vi "Camber controller instrument on-off capability.vi"() -> ()   [LabVIEW 2014]
uses:
  <vilib>/Instr/_visa.llb/VISA Configure Serial Port (Instr).vi
  <vilib>/Utility/file.llb/Write To Spreadsheet File (string).vi
  <vilib>/Utility/file.llb/Read From Spreadsheet File (string).vi
  Environmental Chamber LabVIEW and Instruments/Drivers and Software/Keithley 2100 Series/Public/Configure/Configure 2 Wire Resistance.vi
  Environmental Chamber LabVIEW and Instruments/Drivers and Software/keithley_6430/Keithley 6430/Keithley 6430.lvlib
  Environmental Chamber LabVIEW and Instruments/Drivers and Software/keithley_24xx/Keithley 24XX/Keithley 24XX.lvlib
  Environmental Chamber LabVIEW and Instruments/Drivers and Software/Keithley 2100 Series/Keithley 2100 Series.lvlib
panel:
  out "Arduino QCM freq":T1 caption="Arduino\nQCM freq" {"QCM1" format="%#_8g"; "QCM2" format="%#_8g"; "QCM3" format="%#_8g"; "QCM4" format="%#_8g"; "QCM5" format="%#_8g"}
  in  "Stop":bool
  out "Currently saving data":bool
  in  "Tab Control":T2(tab)
  in  "Instrument Addresses":T3={"J-KEM"="COM3", "Keithley-6430"="GPIB0::30::INSTR", "Keithley-2420"="GPIB1::24::INSTR", "Keithley-2100"="K-2100", "SRS-QCM200"="COM6", "ArduinoQCM1"="COM21", "ArduinoQCM2"="COM22", "ArduinoQCM3"="COM23", "ArduinoQCM4"="COM24", "ArduinoQCM5"="COM26"}
  in  "Instrument on/off":T4
  in  "Data logging settings":T5={"Save during sequence only"=TRUE, "Save now"=FALSE, "seconds between\ndata points"=0.0, "Current data file path"=path "", "Save sample names"={"QCM1"="aQCM2", "QCM2"="aQCM2", "QCM3"="aQCM3", "QCM4"="aQCM4", "QCM5"="aQCM5", "QCM6"="aQCM6", "SRS"="sample_SRS", "K-2420"="Keithley2420", "K-6430"="Keithley6430", "K-2100"="Keithley2100"}, "Experiment Notes"=""} {"seconds between\ndata points" min=0.0 max=30.0 format="%#_13g"}
  out "Sequence\npreview":cluster{dbl[], dbl[]}[](graph) caption="Sequence preview"
  in  "Pressure control cluster":T6={"Save sequence"=FALSE, "Clear sequence"=FALSE, "Import sequence file"=FALSE, "Tare elapsed time"=TRUE, "Run Sequence"=FALSE, "Stop program when sequence ends"=TRUE, "User-defined\nsequence"=[], "Sequence end time"=""} caption="Sequence settings"
  in  "Pressure parameters cluster":T7={"valve % open"=100.0, "Desired pressure"=0.0, "Vapor sccm"=0.0, "Gas sccm"=0.0, "Valve mode"=enum."% Open", "Pressure Mode"=enum."Abs. pressure", "analyte partial pressure"=100.0, "Turbo pump\nauto on"=TRUE, "Valve position (%)"=0.0, "read pressure"=0.0, "read vapor flow"=0.0, "read gas flow"=0.0} caption="Pressure settings" {"read gas flow" format="%#_3g"; "read vapor flow" format="%#_3g"; "read pressure" format="%#_7f"; "Valve position (%)" format="%#_3g"; "analyte partial pressure" min=0.0 max=100.0 step=5.0; "Gas sccm" min=0 max=200 step=5; "Vapor sccm" min=0 max=200 step=5; "Desired pressure" min=0.0 max=760.0 step=5.0; "valve % open" min=0.0 max=100.0 step=5.0 format="%#_2f"}
  out "Pressure chart":dbl(graph)
  out "Temp chart":dbl(graph)
  in  "SRS cluster":T8={"QCM plot"={"Numeric Control"=0.0, "Resistance out"=0.0}, "Gate time (sec)"=1, "Freq (MHz)"=0.0, "Tare mass"=FALSE} caption="SRS QCM" {"Freq (MHz)" format="%.6f"; "Gate time (sec)" items=["0.1 seconds", "1.0 seconds", "10.0 seconds"]}
  out "Keithley charts cluster":T9 caption="Keithley measurements"
  in  "Clear all charts":bool
  out "Elapsed time (min)":dbl
  out "State date/time":string caption="Start time"
  out "Arduino QCM plots":T10 caption="Arduino/OpenQCM"
  # "100%"
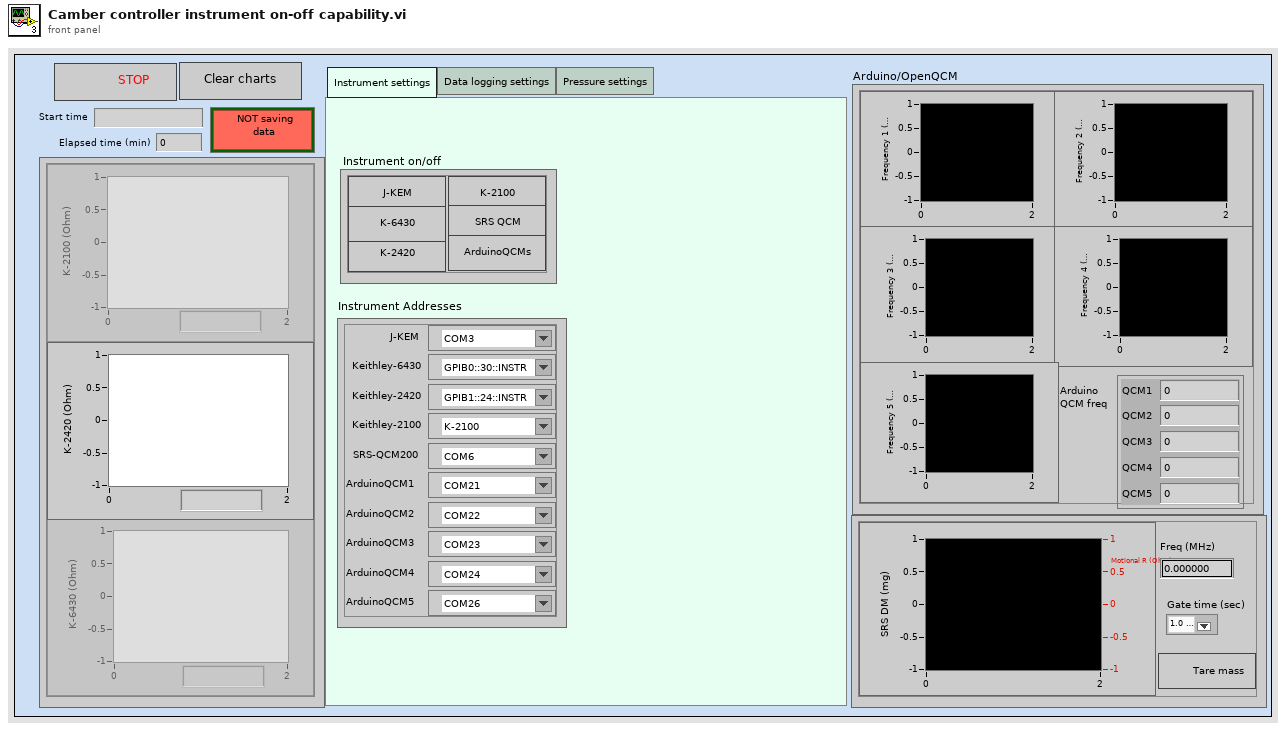
[diagram p1: front panel]
types:
  T1 = cluster{"QCM1":dbl, "QCM2":dbl, "QCM3":dbl, "QCM4":dbl, "QCM5":dbl}
  T2 = enum32{"Instrument settings", "Data logging settings", "Pressure settings"}
  T3 = cluster{"J-KEM":refnum<visa-resource-name>, "Keithley-6430":refnum<visa-resource-name>, "Keithley-2420":refnum<visa-resource-name>, "Keithley-2100":refnum<visa-resource-name>, "SRS-QCM200":refnum<visa-resource-name>, "ArduinoQCM1":refnum<visa-resource-name>, "ArduinoQCM2":refnum<visa-resource-name>, "ArduinoQCM3":refnum<visa-resource-name>, "ArduinoQCM4":refnum<visa-resource-name>, "ArduinoQCM5":refnum<visa-resource-name>}
  T4 = cluster{"J-KEM":bool, "K-2420":bool, "K-2100":bool, "SRS QCM":bool, "ArduiunoQCMs":bool, "K-6430":bool}
  T5 = cluster{"Save during sequence only":bool, "Save now":bool, "seconds between\ndata points":dbl, "Current data file path":path, "Save sample names":cluster{"QCM1":string, "QCM2":string, "QCM3":string, "QCM4":string, "QCM5":string, "QCM6":string, "SRS":string, "K-2420":string, "K-6430":string, "K-2100":string}, "Experiment Notes":string}
  T6 = cluster{"Save sequence":bool, "Clear sequence":bool, "Import sequence file":bool, "Tare elapsed time":bool, "Run Sequence":bool, "Stop program when sequence ends":bool, "User-defined\nsequence":string[][], "Sequence end time":string}
  T7 = cluster{"valve % open":dbl, "Desired pressure":dbl, "Vapor sccm":sgl, "Gas sccm":sgl, "Valve mode":enum32{"% Open", "Torr "}, "Pressure Mode":enum32{"Abs. pressure", " Part. pressure"}, "analyte partial pressure":dbl, "Turbo pump\nauto on":bool, "Valve position (%)":dbl, "read pressure":dbl, "read vapor flow":dbl, "read gas flow":dbl}
  T8 = cluster{"QCM plot":cluster{"Numeric Control":dbl, "Resistance out":dbl}, "Gate time (sec)":u16, "Freq (MHz)":dbl, "Tare mass":bool}
  T9 = cluster{"K-6430 Ohms":dbl, "K-2420 Ohms":sgl, "K-2100 Ohms":dbl}
  T10 = cluster{"arduino qcm 1":dbl, "arduino qcm 2":dbl, "arduino qcm 3":dbl, "arduino qcm 4":dbl, "arduino qcm 5":dbl}
  T11 = enum16{"open", "open or create", "create or replace", "create", "open (read only)"}
  T12 = cluster{"J-KEM":bool, "K-6430":bool, "K-2420":bool, "K-2100":bool, "SRS QCM":bool, "OpenQCMs":bool}
  T13 = enum8{"Enabled", "Disabled", "Disabled and Grayed Out"}
  T14 = cluster{"ArduinoQCM1":refnum<visa-resource-name>, "error out":errorcluster, "ArduinoQCM2":refnum<visa-resource-name>, "error out":errorcluster, "ArduinoQCM3":refnum<visa-resource-name>, "error out":errorcluster, "ArduinoQCM4":refnum<visa-resource-name>, "error out":errorcluster, "ArduinoQCM5":refnum<visa-resource-name>, "error out":errorcluster}
  T15 = cluster{"task out":refnum<k21>, "error out":errorcluster, "task out":refnum<k21>, "error out":errorcluster, "task out":refnum<k21>, "error out":errorcluster, "VISA resource name out":refnum<visa-resource-name>, "error out":errorcluster}
  T16 = cluster{"Turbo\npump":bool, cluster{"task out":refnum<k21>, "error out":errorcluster, "task out":refnum<k21>, "error out":errorcluster, "task out":refnum<k21>, "error out":errorcluster, "VISA resource name out":refnum<visa-resource-name>, "error out":errorcluster}}
  T17 = cluster{"J-KEM":refnum<visa-resource-name>, "error out":errorcluster, "Boolean":bool}
  T18 = cluster{"Keithley-6430":refnum<visa-resource-name>, "error out":errorcluster, "Boolean":bool}
  T19 = cluster{"Keithley-2420":refnum<visa-resource-name>, "error out":errorcluster, "Boolean":bool}
  T20 = cluster{"Keithley-2100":refnum<visa-resource-name>, "error out":errorcluster, "Boolean":bool}
  T21 = cluster{"SRS-QCM200":refnum<visa-resource-name>, "error out":errorcluster, "Boolean":bool}
  T22 = cluster{"Boolean":bool, cluster{"ArduinoQCM1":refnum<visa-resource-name>, "error out":errorcluster, "ArduinoQCM2":refnum<visa-resource-name>, "error out":errorcluster, "ArduinoQCM3":refnum<visa-resource-name>, "error out":errorcluster, "ArduinoQCM4":refnum<visa-resource-name>, "error out":errorcluster, "ArduinoQCM5":refnum<visa-resource-name>, "error out":errorcluster}}
  T23 = cluster{"f":dbl, "f":dbl, "f":dbl, "f":dbl, "f":dbl}
  T24 = cluster{"arduinos on/off":bool, "arduino 1-6 address and errors":cluster{"VISA resource name out":refnum<visa-resource-name>, "error out":errorcluster, "VISA resource name out":refnum<visa-resource-name>, "error out":errorcluster, "VISA resource name out":refnum<visa-resource-name>, "error out":errorcluster, "VISA resource name out":refnum<visa-resource-name>, "error out":errorcluster, "VISA resource name out":refnum<visa-resource-name>, "error out":errorcluster}}
  T25 = cluster{"VISA resource name out":refnum<visa-resource-name>, "error out":errorcluster, "Boolean":bool}
  T26 = cluster{"VISA resource name out":refnum<visa-resource-name>, "error out":errorcluster, "VISA resource name out":refnum<visa-resource-name>, "error out":errorcluster, "VISA resource name out":refnum<visa-resource-name>, "error out":errorcluster, "VISA resource name out":refnum<visa-resource-name>, "error out":errorcluster, "VISA resource name out":refnum<visa-resource-name>, "error out":errorcluster}
  T27 = cluster{"VISA Refnum out":refnum<visa-resource-name>, "error out":errorcluster, "VISA Refnum out":refnum<visa-resource-name>, "error out":errorcluster, "VISA Refnum out":refnum<visa-resource-name>, "error out":errorcluster, "VISA Refnum out":refnum<visa-resource-name>, "error out":errorcluster, "VISA Refnum out":refnum<visa-resource-name>, "error out":errorcluster}
  T28 = cluster{"f":string, "f":string, "f":string, "f":string, "f":string}
  T29 = cluster{"VISA out":refnum<visa-resource-name>, "error out":errorcluster, "Boolean":bool}
  T30 = cluster{"Numeric Control":dbl, "Resistance out":dbl}
  T31 = cluster{"mass_ug":string, "freq_Hz":string, "motional_resistance_Ohm":string}
  T32 = cluster{"K6430 Measurement":dbl, "Resistance":sgl, "Measurement":dbl}
  T33 = cluster{"arduinos on? output":bool, "arduino 1-6 addresses and errors out":cluster{"VISA Refnum out":refnum<visa-resource-name>, "error out":errorcluster, "VISA Refnum out":refnum<visa-resource-name>, "error out":errorcluster, "VISA Refnum out":refnum<visa-resource-name>, "error out":errorcluster, "VISA Refnum out":refnum<visa-resource-name>, "error out":errorcluster, "VISA Refnum out":refnum<visa-resource-name>, "error out":errorcluster}}
  T34 = cluster{"String data out":string, "K6430 measuremnet string":string, "String":string, "String":string}
  T35 = cluster{"VISA resource name out":refnum<visa-resource-name>, "error out":errorcluster, bool}
  T36 = cluster{"VISA out":refnum<visa-resource-name>, "error out":errorcluster, bool}
  T37 = cluster{"VISA resource name out":refnum<visa-resource-name>, "VISA resource name out":refnum<visa-resource-name>, "VISA resource name out":refnum<visa-resource-name>, "VISA resource name out":refnum<visa-resource-name>, "VISA resource name out":refnum<visa-resource-name>}
  T38 = cluster{"arduinos on/off":bool, "arduino addresses/errors":cluster{"VISA resource name out":refnum<visa-resource-name>, "error out":errorcluster, "VISA resource name out":refnum<visa-resource-name>, "error out":errorcluster, "VISA resource name out":refnum<visa-resource-name>, "error out":errorcluster, "VISA resource name out":refnum<visa-resource-name>, "error out":errorcluster, "VISA resource name out":refnum<visa-resource-name>, "error out":errorcluster}}
  T39 = cluster{"valve % open":dbl, "Desired pressure":dbl, "Vapor sccm":sgl, "Gas sccm":sgl, "Valve mode":enum32{"% Open", "Torr "}, "Pressure Mode":enum32{"Abs. pressure", " Part. pressure"}, "analyte partial pressure":dbl, "Turbo pump\nauto on":bool}
  T40 = cluster{"User-defined\nsequence":string[][], "Present (s)":dbl, "current  step # in":i32, "sequence end time in":timestamp}
  T41 = cluster{"current  step # in":i32, "sequence end time in":timestamp, "Boolean":bool}
  T42 = cluster{"press/RH/gas/vapor":cluster{"pressure":string, "RH":string, "gas flow":string, "vapor flow":string}, "Cluster":cluster{"Valve position (%)":dbl, "read pressure":dbl, "read vapor flow":dbl, "read gas flow":dbl}}
  T43 = cluster{"Boolean":bool, "DAQ IDs in":cluster{"task out":refnum<k21>, "error out":errorcluster, "task out":refnum<k21>, "error out":errorcluster, "task out":refnum<k21>, "error out":errorcluster, "VISA Refnum out":refnum<visa-resource-name>, "error out":errorcluster}}
  T44 = cluster{"pressure":string, "RH":string, "gas flow":string, "vapor flow":string}
  T45 = cluster{"Valve position (%)":dbl, "read pressure":dbl, "read vapor flow":dbl, "read gas flow":dbl}
  T46 = cluster{"QCM1":string, "QCM2":string, "QCM3":string, "QCM4":string, "QCM5":string, "QCM6":string, "SRS":string, "K-2420":string, "K-6430":string, "K-2100":string}
  T47 = cluster{"task out":refnum<k21>, "error out":errorcluster, "task out":refnum<k21>, "error out":errorcluster, "task out":refnum<k21>, "error out":errorcluster, "VISA Refnum out":refnum<visa-resource-name>, "error out":errorcluster}
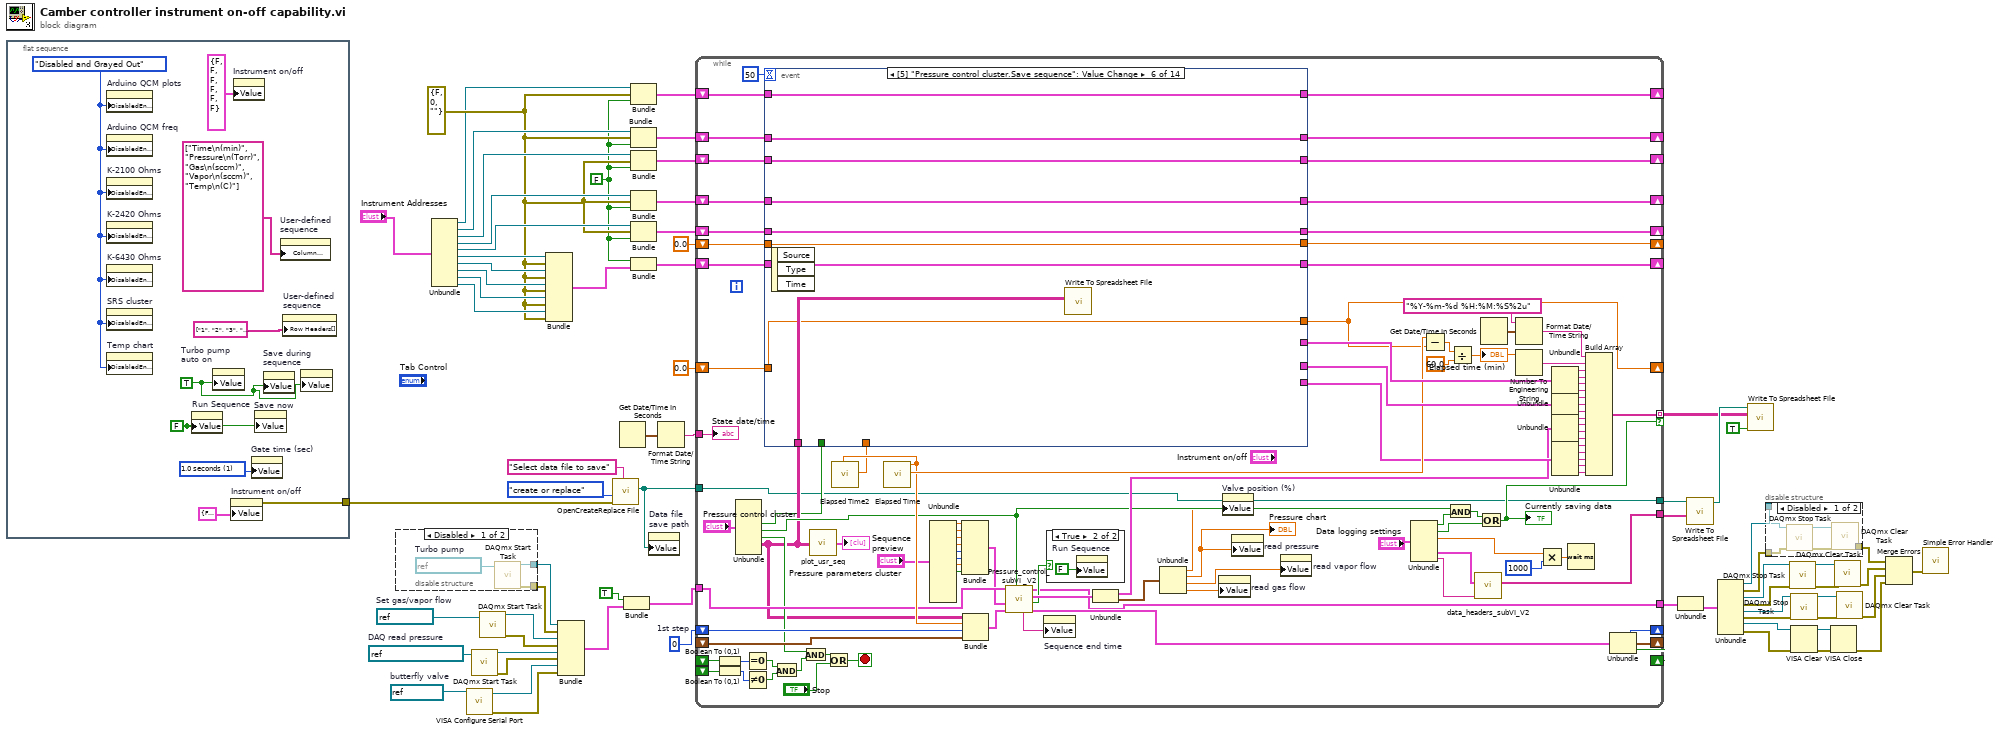
[diagram p0: block diagram]
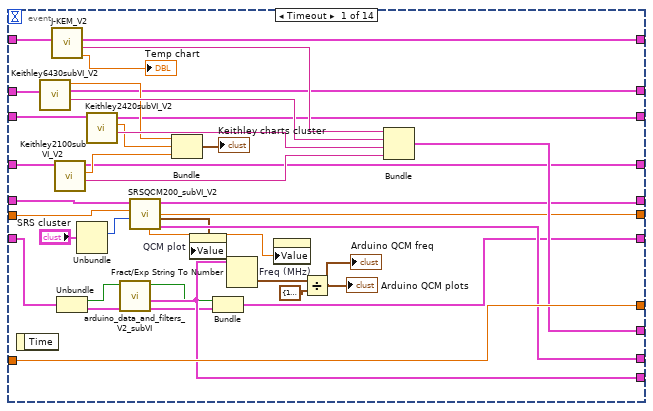
[diagram p5: hidden frame]
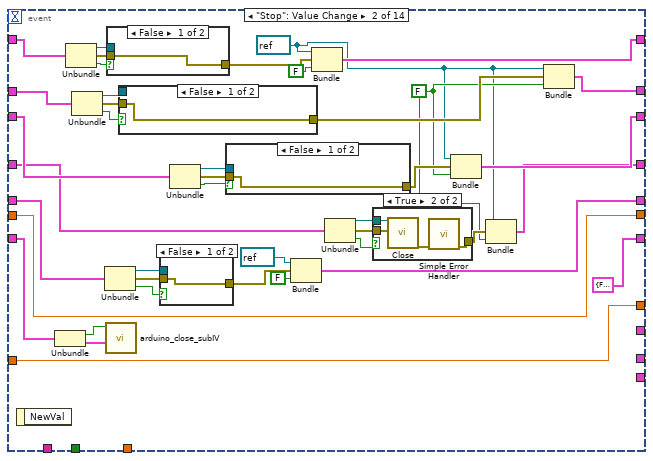
[diagram p6: hidden frame]
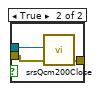
[diagram p8: hidden frame]
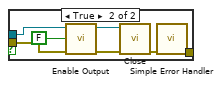
[diagram p9: hidden frame]
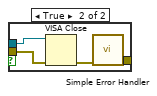
[diagram p10: hidden frame]
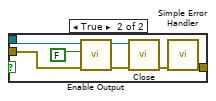
[diagram p11: hidden frame]
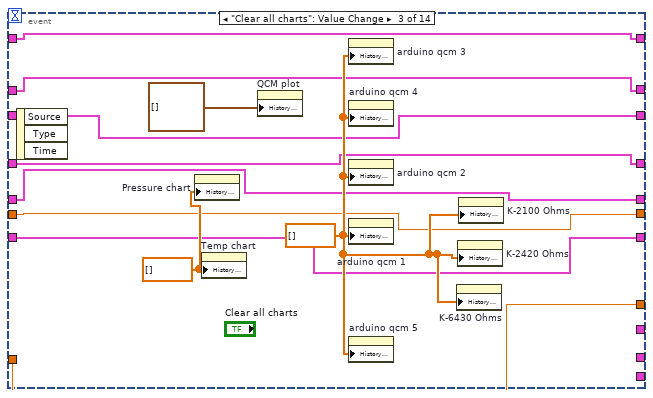
[diagram p12: hidden frame]
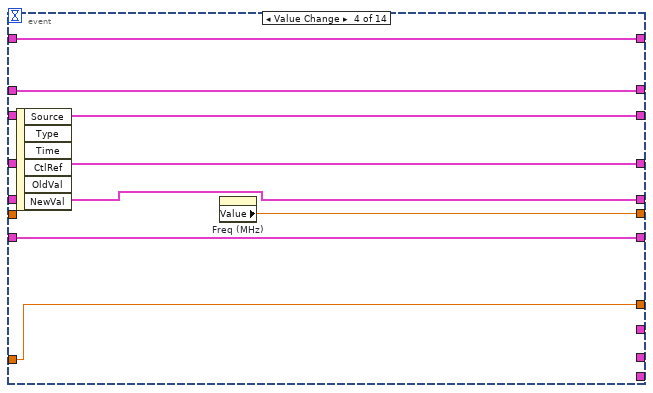
[diagram p13: hidden frame]
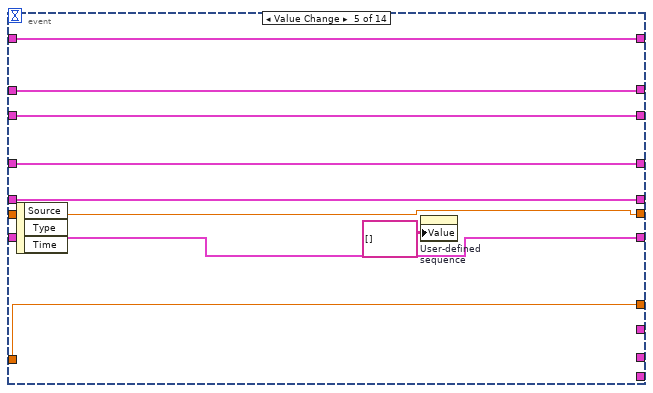
[diagram p14: hidden frame]
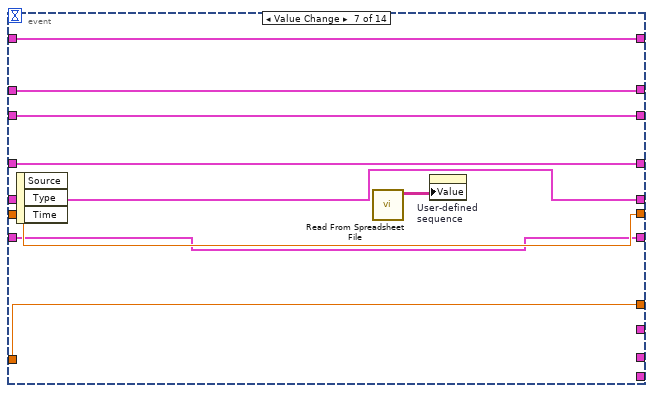
[diagram p15: hidden frame]
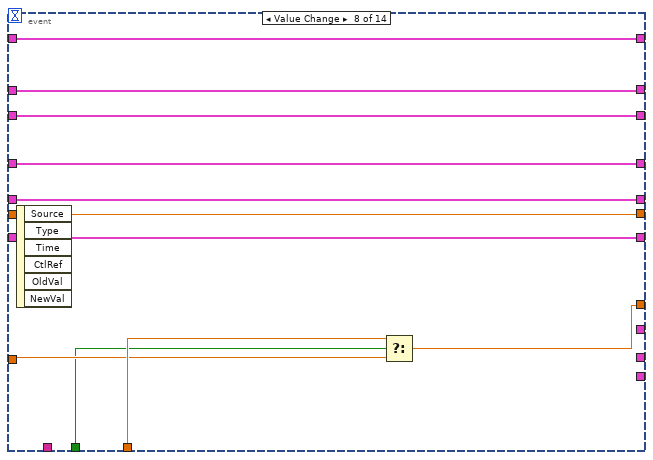
[diagram p16: hidden frame]
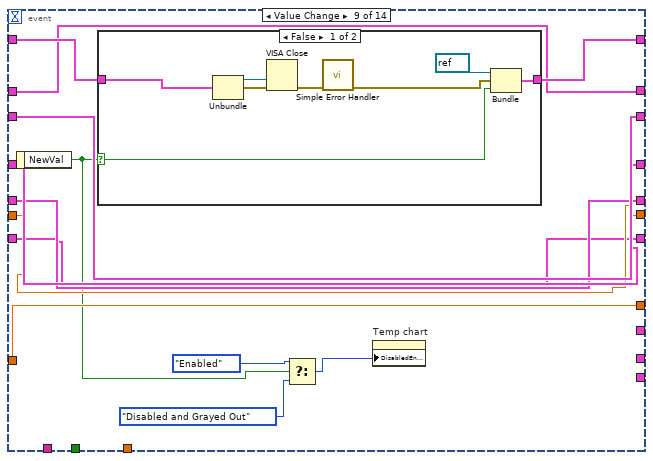
[diagram p17: hidden frame]
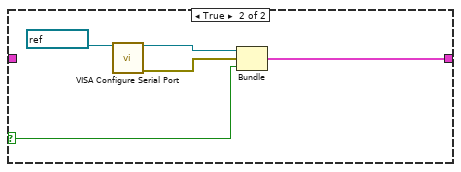
[diagram p18: hidden frame]
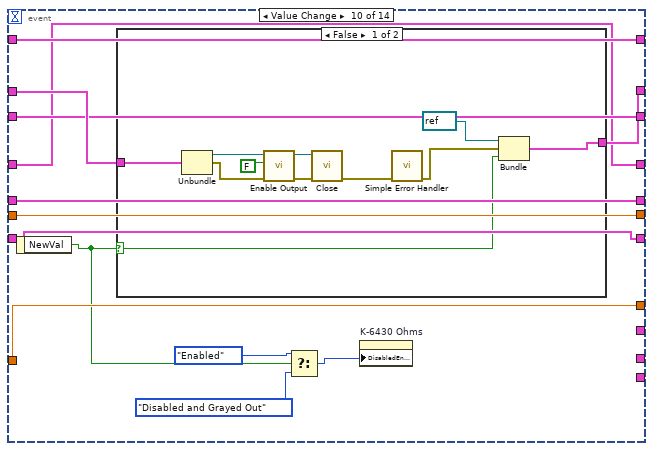
[diagram p19: hidden frame]
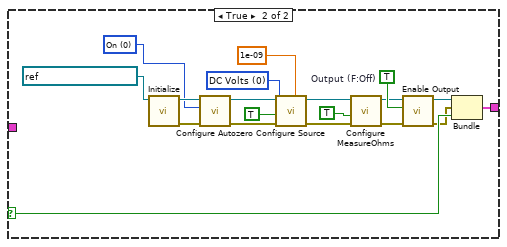
[diagram p20: hidden frame]
diagram:
  w5 = errorcluster {"status"=FALSE, "code"=0, "source"=""} ("error out")
  w4 = FALSE ("Boolean")
  w34 = refnum<visa-resource-name> "COM5"  # butterfly valve
  w35 = refnum<k21> "Setflow"  # Set gas/vapor flow
  w36 = refnum<k21> "AllDaqReadings"  # DAQ read pressure
  w64 = 0  # 1st step
  n1 = flat-sequence {
    tunnel: [w73] -> w56
    frame #0 {
      w71 = T13."Disabled and Grayed Out" ("Disabled")
      w76 = u16 1 items=["0.1 seconds", "1.0 seconds", "10.0 seconds"] ("Gate time")
      w77 = FALSE ("Run Sequence")
      w75 = TRUE ("Turbo\npump")
      n2 = property on="Arduino QCM plots" class="Clust (strict)"("DisabledEnum"=w71) -> ()  [unwired: 2 in, 2 out]
      n3 = property on="Arduino QCM freq" class="Clust (strict)"("DisabledEnum"=w71) -> ()  [unwired: 2 in, 2 out]
      n4 = property on="K-2100 Ohms" class="WFChart (strict)"("DisabledEnum"=w71) -> ()  [unwired: 2 in, 2 out]
      n5 = property on="K-2420 Ohms" class="WFChart (strict)"("DisabledEnum"=w71) -> ()  [unwired: 2 in, 2 out]
      n6 = property on="K-6430 Ohms" class="WFChart (strict)"("DisabledEnum"=w71) -> ()  [unwired: 2 in, 2 out]
      n7 = property on="SRS cluster" class="Clust"("DisabledEnum"=w71) -> ()  [unwired: 2 in, 2 out]
      n8 = property on="Temp chart" class="WFChart (strict)"("DisabledEnum"=w71) -> ()  [unwired: 2 in, 2 out]
      n9 = property on="Run Sequence" class="Bool (strict)"("Value"=w77) -> ()  [unwired: 2 in, 2 out]
      n10 = property on="Turbo pump\nauto on" class="Bool (strict)"("Value"=w75) -> ()  [unwired: 2 in, 2 out]
      n11 = property on="Instrument on/off" class="Clust (strict)"("Value"=T12 {"J-KEM"=FALSE, "K-6430"=FALSE, "K-2420"=FALSE, "K-2100"=FALSE, "SRS QCM"=FALSE, "OpenQCMs"=FALSE} ("Instrument on/off")) -> (error out=w73:errorcluster)  [unwired: 2 in, 1 out]
      n12 = property on="Instrument on/off" class="Clust (strict)"("Value"=T4 {"J-KEM"=FALSE, "K-2420"=FALSE, "K-2100"=FALSE, "SRS QCM"=FALSE, "ArduiunoQCMs"=FALSE, "K-6430"=FALSE} ("Instrument on/off")) -> ()  [unwired: 2 in, 2 out]
      n13 = property on="Gate time (sec)" class="Ring (strict)"("Value"=w76) -> ()  [unwired: 2 in, 2 out]
      n14 = property on="Save now" class="Bool (strict)"("Value"=w77) -> ()  [unwired: 2 in, 2 out]
      n15 = property on="Save during\nsequence" class="Bool (strict)"("Value"=w75) -> ()  [unwired: 2 in, 2 out]
      n16 = property on="User-defined\nsequence" class="Tbl (strict)"("Column Headers[]"=string[] ["Time\n(min)", "Pressure\n(Torr)", "Gas\n(sccm)", "Vapor\n(sccm)", "Temp\n(C)"] ("Column Header Strings[]")) -> ()  [unwired: 2 in, 2 out]
      n17 = property on="User-defined\nsequence" class="Tbl (strict)"("Row Headers[]"=string[] ["1", "2", "3", "4", "5", "6", "7", "8", "9", "10", "11", "12", "13", "14", "15", "16", "17", "18", "19", "20", "21", "22", "23", "24", "25", "26", "27", "28", "29", "30", "31", "32", "33", "34", "35", "36", "37", "38", "39", "40", "41", "42", "43", "44", "45", "46", "47", "48", "49", "50"] ("Row Header Strings[]")) -> ()  [unwired: 2 in, 2 out]
      n18 = property on="Stop program when sequence ends" class="Bool (strict)"("Value"=w75) -> ()  [unwired: 2 in, 2 out]
    }
  }
  n19 = disable-structure shown="Disabled" {
    disable-tunnel: [w80 _] -> w33
    disable-tunnel: [w79 _] -> w32
    frame Disabled {
      w81 = refnum<k21> "TurboON"  # Turbo pump
      n20 = call <vilib>:"DAQmx Start Task.vi"("task/channels in"=w81) -> ("task out"=w80:refnum<k21>, "error out"=w79:errorcluster)  [unwired: 13 in]
    }
    frame Enabled {
    }
  }
  n21 = Unbundle("Instrument Addresses") -> ("J-KEM"=w3:refnum<visa-resource-name>, "Keithley-6430"=w18:refnum<visa-resource-name>, "Keithley-2420"=w16:refnum<visa-resource-name>, "Keithley-2100"=w14:refnum<visa-resource-name>, "SRS-QCM200"=w12:refnum<visa-resource-name>, "ArduinoQCM1"=w10:refnum<visa-resource-name>, "ArduinoQCM2"=w9:refnum<visa-resource-name>, "ArduinoQCM3"=w8:refnum<visa-resource-name>, "ArduinoQCM4"=w7:refnum<visa-resource-name>, "ArduinoQCM5"=w6:refnum<visa-resource-name>)
  n22 = call-poly "VISA Configure Serial Port"("VISA resource name"=w34) -> ("VISA resource name out"=w27:refnum<visa-resource-name>, "error out"=w26:errorcluster)  [unwired: 13 in]
  n23 = call <vilib>:"DAQmx Start Task.vi"("task/channels in"=w36) -> ("task out"=w29:refnum<k21>, "error out"=w28:errorcluster)  [unwired: 13 in]
  n24 = call <vilib>:"DAQmx Start Task.vi"("task/channels in"=w35) -> ("task out"=w31:refnum<k21>, "error out"=w30:errorcluster)  [unwired: 13 in]
  n25 = Bundle("ArduinoQCM1"=w10, "error out"=w5, "ArduinoQCM2"=w9, "error out"=w5, "ArduinoQCM3"=w8, "error out"=w5, "ArduinoQCM4"=w7, "error out"=w5, "ArduinoQCM5"=w6, "error out"=w5) -> (w1:T14)  [unwired: 1 in]
  n26 = Bundle("task out"=w33, "error out"=w32, "task out"=w31, "error out"=w30, "task out"=w29, "error out"=w28, "VISA resource name out"=w27, "error out"=w26) -> (w21:T15)  [unwired: 1 in]
  n27 = call "OpenCreateReplace File.vi"("prompt"="Select data file to save", "error in (no error)"=w56, "function (open:0)"=T11."create or replace") -> ("new file path"=w62:path)  [unwired: 5 in, 3 out]
  n28 = Get Date/Time In Seconds() -> (seconds since 1Jan1904=w69:timestamp)
  n29 = Bundle("Turbo\npump"=TRUE ("Turbo\npump"), w21) -> (w22:T16)  [unwired: 1 in]
  n30 = Bundle("J-KEM"=w3, "error out"=w5, "Boolean"=w4) -> (w19:T17)  [unwired: 1 in]
  n31 = Bundle("Keithley-6430"=w18, "error out"=w5, "Boolean"=w4) -> (w17:T18)  [unwired: 1 in]
  n32 = Bundle("Keithley-2420"=w16, "error out"=w5, "Boolean"=w4) -> (w15:T19)  [unwired: 1 in]
  n33 = Bundle("Keithley-2100"=w14, "error out"=w5, "Boolean"=w4) -> (w13:T20)  [unwired: 1 in]
  n34 = Bundle("SRS-QCM200"=w12, "error out"=w5, "Boolean"=w4) -> (w11:T21)  [unwired: 1 in]
  n35 = Bundle("Boolean"=w4, w1) -> (w2:T22)  [unwired: 1 in]
  n36 = property on="Data file\nsave path" class="Path"("Value"=w62) -> ()  [unwired: 2 in, 2 out]
  n37 = Format Date/Time String(seconds (now)=w69) -> (date/time string=w60:string)  [unwired: 2 in]
  n38 = while {
    tunnel: [w82] -> w65
    tunnel: w62 -> [w82]
    shift-right: [w123] -> _
    shift-left: w64 -> [w125]
    shift-right: [w122] -> _
    shift-left: _ -> [w126]
    tunnel: [w182] -> w63
    shift-right: [w121] -> _
    shift-left: _ -> [w181]
    shift-left: _ -> [w180]
    shift-right: [w95] -> _
    shift-left: 0.0 ("Elapsed Time (s)") -> [w96]
    tunnel: w60 -> [w167]
    shift-right: [w166] -> _
    shift-left: w19 -> [w165]
    shift-right: [w163] -> _
    shift-left: w17 -> [w162]
    shift-right: [w161] -> _
    shift-left: w15 -> [w160]
    shift-right: [w159] -> _
    shift-left: w13 -> [w158]
    shift-right: [w156] -> _
    shift-left: w11 -> [w157]
    shift-right: [w155] -> _
    shift-left: 0.0 ("Frequency out 3") -> [w154]
    tunnel: [w141] -> w58 mode=indexing if=w91
    shift-right: [w131] -> _
    shift-left: w2 -> [w130]
    tunnel: w22 -> [w116]
    tunnel: [w115] -> w25
    stop <- w173 stop-if-true
    n39 = Boolean To (0,1)(Boolean=w181) -> (0, 1=w179:i16)
    n40 = Boolean To (0,1)(Boolean=w180) -> (0, 1=w178:i16)
    n41 = Unbundle("Pressure control cluster") -> ("Tare elapsed time"=w94:bool, "Run Sequence"=w113:bool, "Stop program when sequence ends"=w114:bool, "User-defined\nsequence"=w112:string[][])  [unwired: 4 out]
    n42 = Equal To 0?(x=w179) -> (x = 0?=w176:bool)
    n43 = Not Equal To 0?(x=w178) -> (x != 0?=w177:bool)
    n44 = And(x=w176, y=w177) -> (x .and. y?=w172:bool)
    n45 = And(x=w114, y=w172) -> (x .and. y?=w169:bool)
    n46 = call "plot_usr_seq.vi"("User-defined sequence"=w112) -> ("Sequence Preview"=→"Sequence\npreview":cluster{dbl[], dbl[]}[])
    n47 = Or(x=w169, y="Stop") -> (x .or. y?=w173:bool)
    n48 = call "Elapsed Time"() -> ("Present (s)"=w128:dbl, "Elapsed Time (s)"=w142:dbl)  [unwired: 12 in, 6 out]
    n49 = call "Elapsed Time2"("Set Start Time (s)"=w128) -> ("Elapsed Time (s)"=w97:dbl)  [unwired: 11 in, 7 out]
    n50 = event shown="[5] \"Pressure control cluster.Save sequence\": Value Change" {
      selector: _ -> [_ _ _ _ _ _ _ _ _ _ _ _ _ _]
      dyn-events: _ -> [_ _ _ _ _ _ _ _ _ _ _ _ _ _]
      timeout: 50 -> [_ _ _ _ _ _ _ _ _ _ _ _ _ _]
      tunnel: [w193 w260 w303 w313 w322 w331 w340 w348 w365 w389 w432 w473 w502 w524] -> w166
      tunnel: w165 -> [w224 w261 w303 w313 w322 w331 w340 w348 w364 w389 w432 w473 w502 w524]
      tunnel: w162 -> [w223 w255 w302 w312 w321 w330 w339 w347 w363 w391 w431 w472 w501 w523]
      tunnel: [w192 w251 w302 w312 w321 w330 w339 w347 w363 w390 w431 w472 w501 w523] -> w163
      tunnel: [w191 w249 w301 w311 w320 w329 w338 w346 w362 w388 w434 w474 w500 w522] -> w161
      tunnel: w160 -> [w222 w252 w301 w311 w320 w329 w338 w346 w362 w388 w433 _ w500 w522]
      tunnel: w158 -> [w221 w245 w300 w310 w319 w328 w337 w345 w361 w387 w430 w475 w499 w521]
      tunnel: [w188 w237 w300 w310 w319 w328 w337 w345 w361 w387 w430 w475 w499 w521] -> w159
      tunnel: w157 -> [w220 w240 w299 w309 w318 w327 w336 w344 w360 w386 w429 w471 w504 w520]
      tunnel: [w189 w238 w299 w309 w318 w327 w336 w344 w360 w386 w429 w471 w503 w520] -> w156
      tunnel: [w190 w265 w298 w314 w317 w326 w335 w343 w359 w385 w428 w470 w496 w519] -> w155
      tunnel: w154 -> [w219 w265 w298 _ w317 w326 w335 w343 w359 w385 w428 w470 w496 w519]
      tunnel: w97 -> [_ _ _ _ _ _ _ w352 _ _ _ _ _ _]
      tunnel: w96 -> [w218 w229 w296 w307 w315 w324 w333 w351 w357 w383 w426 w468 w497 w518]
      tunnel: [w218 w229 w296 w307 w315 w324 w333 w350 w357 w383 w426 w468 w497 w518] -> w95
      tunnel: w112 -> [_ _ _ _ _ w332 _ _ _ _ _ _ _ _]
      tunnel: [w214 _ _ _ _ _ _ _ _ _ _ _ _ _] -> w147
      tunnel: [w213 _ _ _ _ _ _ _ _ _ _ _ _ _] -> w146
      tunnel: [w203 T24 {"arduinos on/off"=FALSE, "arduino 1-6 address and errors"={"VISA resource name out"="", "error out"={"status"=FALSE, "code"=0, "source"=""}, "VISA resource name out"="", "error out"={"status"=FALSE, "code"=0, "source"=""}, "VISA resource name out"="", "error out"={"status"=FALSE, "code"=0, "source"=""}, "VISA resource name out"="", "error out"={"status"=FALSE, "code"=0, "source"=""}, "VISA resource name out"="", "error out"={"status"=FALSE, "code"=0, "source"=""}}} w297 w308 w316 w325 w334 w342 w358 w384 w427 w469 w498 w530] -> w131
      tunnel: w130 -> [w209 w234 w297 w308 w316 w325 w334 w342 w358 w384 w427 w469 w498 w529]
      tunnel: [w206 _ _ _ _ _ _ _ _ _ _ _ _ _] -> w129
      tunnel: w94 -> [_ _ _ _ _ _ _ w349 _ _ _ _ _ _]
      event Timeout {
        n51 = event-data() -> ()  [unwired: 1 in, 1 out]
        n52 = call "Keithley6430subVI_V2.vi"("K-6430 info in"=w223) -> ("K6430 Measurement"=w202:dbl, "K6430 info out"=w192:T25, "K6430 measuremnet string"=w216:string)  [unwired: 7 in]
        n53 = call "J-KEM_V2.vi"("info in"=w224) -> ("Temp (C)"=→"Temp chart":dbl, "String data out"=w217:string, "info out"=w193:T25)  [unwired: 7 in, 1 out]
        n54 = call "Keithley2100subVI_V2.vi"("K-2100 init"=w221) -> ("String"=w212:string, "Measurement"=w199:dbl, "Cluster"=w188:T25)  [unwired: 8 in]
        n55 = Unbundle(w209) -> ("arduinos on/off"=w208:bool, "arduino addresses/errors"=w207:T26)
        n56 = Unbundle("SRS cluster") -> ("Gate time (sec)"=w197:u16)  [unwired: 3 out]
        n57 = call "Keithley2420subVI_V2.vi"("K-2420 init"=w222) -> ("String"=w215:string, "Resistance"=w201:sgl, "Cluster"=w191:T25)  [unwired: 8 in]
        n58 = call "arduino_data_and_filters_V2_subVI.vi"("arduino 1-6 address and errors"=w207, "arduinos on?"=w208) -> ("arduino 1-6 addresses and errors out"=w205:T27, "arduino 1-6 data out"=w206:T28, "arduinos on? output"=w204:bool)  [unwired: 7 in]
        n59 = call "SRSQCM200_subVI_V2.vi"("SRS QCM init"=w220, "Frequency in"=w219, "Gate time"=w197) -> ("Numeric Control out"=w196:dbl, "info out"=w189:T29, "Frequency out 3"=w190:dbl, "plot freq"=w195:T30, "M,F,MR output cluster"=w213:T31)  [unwired: 3 in]
        n60 = Bundle("K6430 Measurement"=w202, "Resistance"=w201, "Measurement"=w199) -> (→"Keithley charts cluster":T32)  [unwired: 1 in]
        n61 = property on="QCM plot" class="WFChart (strict)"("Value"=w195) -> ()  [unwired: 2 in, 2 out]
        n62 = Bundle("arduinos on? output"=w204, "arduino 1-6 addresses and errors out"=w205) -> (w203:T33)  [unwired: 1 in]
        n63 = Fract/Exp String To Number(string=w206) -> (number=w210:T23)  [unwired: 3 in, 1 out]
        n64 = property on="Freq (MHz)" class="DigNum (strict)"("Value"=w196) -> ()  [unwired: 2 in, 2 out]
        n65 = Divide(x=w210, y=T23 {"f"=1000000.0, "f"=1000000.0, "f"=1000000.0, "f"=1000000.0, "f"=1000000.0}) -> (x/y=→"Arduino QCM plots" →"Arduino QCM freq":T23)
        n66 = Bundle("String data out"=w217, "K6430 measuremnet string"=w216, "String"=w215, "String"=w212) -> (w214:T34)  [unwired: 1 in]
      }
      event "Stop": Value Change {
        w226 = FALSE ("Boolean")
        w225 = refnum<visa-resource-name> refnum ("VISA resource name out")
        n67 = event-data() -> ()  [unwired: 1 in, 1 out]
        n68 = Unbundle(w234) -> ("arduinos on/off"=w236:bool, "arduino addresses/errors"=w235:T26)
        n69 = Unbundle(w261) -> ("J-KEM"=w264:refnum<visa-resource-name>, "error out"=w263:errorcluster, "Boolean"=w231:bool)
        n70 = Unbundle(w255) -> ("Keithley-6430"=w256:refnum<visa-resource-name>, "error out"=w257:errorcluster, "Boolean"=w232:bool)
        n71 = Unbundle(w240) -> ("SRS-QCM200"=w244:refnum<visa-resource-name>, "error out"=w241:errorcluster, "Boolean"=w228:bool)
        n72 = call "arduino_close_subIV.vi"("arduino 1-6 addresses and errors out"=w235, "arduinos on?"=w236) -> ()  [unwired: 10 in]
        n73 = case shown="False" w231 {
          tunnel: w264 -> [_ w287]
          tunnel: w263 -> [w283 w286]
          tunnel: [w283 w284] -> w262
          frame False {
          }
          frame True {
            n74 = VISA Close(VISA resource name=w287, error in (no error)=w286) -> (error out=w285:errorcluster)
            n75 = call <vilib>:"Simple Error Handler.vi"("error in (no error)"=w285) -> ("error out"=w284:errorcluster)  [unwired: 4 in, 4 out]
          }
        }
        n76 = case shown="False" w232 {
          tunnel: [w288 w294] -> w258
          tunnel: w257 -> [w288 w293]
          tunnel: w256 -> [_ w292]
          frame False {
          }
          frame True {
            n77 = call "Enable Output.vi"("error in (no error)"=w293, "Enable Output (F:Off)"=FALSE ("Output (F:Off)"), "VISA resource name"=w292) -> ("error out"=w291:errorcluster, "VISA resource name out"=w290:refnum<visa-resource-name>)  [unwired: 7 out]
            n78 = call "Close.vi"("error in (no error)"=w291, "VISA resource name"=w290) -> ("error out"=w295:errorcluster)  [unwired: 9 out]
            n79 = call <vilib>:"Simple Error Handler.vi"("error in (no error)"=w295) -> ("error out"=w294:errorcluster)  [unwired: 4 in, 4 out]
          }
        }
        n80 = case shown="False" w228 {
          tunnel: w244 -> [_ w274]
          tunnel: [w271 w273] -> w243
          tunnel: w241 -> [w271 w272]
          frame False {
          }
          frame True {
            n81 = call "srsQcm200Close.vi"("error in"=w272, "Visa in"=w274) -> ("error out"=w273:errorcluster)  [unwired: 3 in]
          }
        }
        n82 = Unbundle(w252) -> ("Keithley-2420"=w250:refnum<visa-resource-name>, "error out"=w254:errorcluster, "Boolean"=w230:bool)
        n83 = case shown="False" w230 {
          tunnel: w254 -> [w275 w280]
          tunnel: [w275 w278] -> w253
          tunnel: w250 -> [_ w277]
          frame False {
          }
          frame True {
            n84 = call "Enable Output.vi"("error in (no error)"=w280, "Enable Output (T: Enable)"=FALSE, "VISA resource name"=w277) -> ("error out"=w282:errorcluster, "VISA resource name out"=w281:refnum<visa-resource-name>)  [unwired: 7 in]
            n85 = call "Close.vi"("error in (no error)"=w282, "VISA resource name"=w281) -> ("error out"=w279:errorcluster)  [unwired: 9 in]
            n86 = call <vilib>:"Simple Error Handler.vi"("error in (no error)"=w279) -> ("error out"=w278:errorcluster)  [unwired: 4 in, 4 out]
          }
        }
        n87 = Bundle("VISA resource name out"=refnum<visa-resource-name> refnum, "error out"=w243, "Boolean"=FALSE) -> (w238:T25)  [unwired: 1 in]
        n88 = Bundle("VISA resource name out"=w225, "error out"=w262, "Boolean"=FALSE) -> (w260:T25)  [unwired: 1 in]
        n89 = Unbundle(w245) -> ("Keithley-2100"=w248:refnum<visa-resource-name>, "error out"=w247:errorcluster, "Boolean"=w227:bool)
        n90 = case shown="True" w227 {
          tunnel: w248 -> [_ w270]
          tunnel: w247 -> [w266 w269]
          tunnel: [w266 w267] -> w246
          frame False {
          }
          frame True {
            n91 = call "Close.vi"("VISA resource name"=w270, "error in (no error)"=w269) -> ("error out"=w268:errorcluster)  [unwired: 17 in]
            n92 = call <vilib>:"Simple Error Handler.vi"("error in (no error)"=w268) -> ("error out"=w267:errorcluster)  [unwired: 4 in, 4 out]
          }
        }
        n93 = Bundle("VISA resource name out"=w225, "error out"=w253, "Boolean"=w226) -> (w249:T25)  [unwired: 1 in]
        n94 = Bundle("VISA resource name out"=w225, "error out"=w246, "Boolean"=w226) -> (w237:T25)  [unwired: 1 in]
        n95 = Bundle("VISA resource name out"=w225, "error out"=w258, "Boolean"=w226) -> (w251:T25)  [unwired: 1 in]
      }
      event "Clear all charts": Value Change {
        w304 = dbl[] [] ("History Data")
        w306 = dbl[] [] ("History Data")
        n96 = event-data() -> ()  [unwired: 1 in, 3 out]
        n97 = property on="Pressure chart" class="WFChart (strict)"("History Data"=w304) -> ()  [unwired: 2 in, 2 out]
        n98 = property on="Temp chart" class="WFChart (strict)"("History Data"=w304) -> ()  [unwired: 2 in, 2 out]
        n99 = property on="QCM plot" class="WFChart (strict)"("History Data"=cluster{dbl, "Resistance out":dbl}[] []) -> ()  [unwired: 2 in, 2 out]
        n100 = property on="arduino qcm 3" class="WFChart (strict)"("History Data"=w306) -> ()  [unwired: 2 in, 2 out]
        n101 = property on="arduino qcm 4" class="WFChart (strict)"("History Data"=w306) -> ()  [unwired: 2 in, 2 out]
        n102 = property on="arduino qcm 2" class="WFChart (strict)"("History Data"=w306) -> ()  [unwired: 2 in, 2 out]
        n103 = property on="arduino qcm 1" class="WFChart (strict)"("History Data"=w306) -> ()  [unwired: 2 in, 2 out]
        n104 = property on="arduino qcm 5" class="WFChart (strict)"("History Data"=w306) -> ()  [unwired: 2 in, 2 out]
        n105 = property on="K-6430 Ohms" class="WFChart (strict)"("History Data"=w306) -> ()  [unwired: 2 in, 2 out]
        n106 = property on="K-2420 Ohms" class="WFChart (strict)"("History Data"=w306) -> ()  [unwired: 2 in, 2 out]
        n107 = property on="K-2100 Ohms" class="WFChart (strict)"("History Data"=w306) -> ()  [unwired: 2 in, 2 out]
      }
      event "SRS cluster.Tare mass": Value Change {
        n108 = event-data() -> ()  [unwired: 1 in, 6 out]
        n109 = property on="Freq (MHz)" class="DigNum (strict)"() -> ("Value"=w314:dbl)  [unwired: 2 in, 2 out]
      }
      event "Pressure control cluster.Clear sequence": Value Change {
        n110 = event-data() -> ()  [unwired: 1 in, 3 out]
        n111 = property on="User-defined\nsequence" class="Tbl (strict)"("Value"=string[][] []) -> ()  [unwired: 2 in, 2 out]
      }
      event "Pressure control cluster.Save sequence": Value Change {
        n112 = event-data() -> ()  [unwired: 1 in, 3 out]
        n113 = call-poly <vilib>:"Write To Spreadsheet File.vi"("2D data"=w332) -> ()  [unwired: 7 in, 1 out]
      }
      event "Pressure control cluster.Import sequence file": Value Change {
        n114 = event-data() -> ()  [unwired: 1 in, 3 out]
        n115 = call-poly <vilib>:"Read From Spreadsheet File.vi"() -> ("all rows"=w341:string[][])  [unwired: 7 in, 4 out]
        n116 = property on="User-defined\nsequence" class="Tbl (strict)"("Value"=w341) -> ()  [unwired: 2 in, 2 out]
      }
      event "Pressure control cluster.Run Sequence": Value Change {
        n117 = event-data() -> ()  [unwired: 1 in, 6 out]
        n118 = Select(t=w352, s=w349, f=w351) -> (s? t:f=w350:dbl)
      }
      event "Instrument on/off.J-KEM": Value Change {
        n119 = event-data() -> ("NewVal"=w354:bool)  [unwired: 1 in]
        n120 = case shown="False" w354 {
          selector: w354 -> [w369 w375]
          tunnel: [w367 w376] -> w365
          tunnel: w364 -> [w373 _]
          frame False {
            n121 = Unbundle(w373) -> ("J-KEM"=w372:refnum<visa-resource-name>, "error out"=w371:errorcluster)  [unwired: 1 out]
            n122 = VISA Close(VISA resource name=w372, error in (no error)=w371) -> (error out=w370:errorcluster)
            n123 = call <vilib>:"Simple Error Handler.vi"("error in (no error)"=w370) -> ("error out"=w366:errorcluster)  [unwired: 4 in, 4 out]
            n124 = Bundle("VISA resource name out"=refnum<visa-resource-name> refnum, "error out"=w366, w369) -> (w367:T35)  [unwired: 1 in]
          }
          frame True {
            n125 = call-poly "VISA Configure Serial Port"("VISA resource name"=refnum<visa-resource-name> "COM3") -> ("VISA resource name out"=w378:refnum<visa-resource-name>, "error out"=w374:errorcluster)  [unwired: 13 in]
            n126 = Bundle("VISA resource name out"=w378, "error out"=w374, w375) -> (w376:T35)  [unwired: 1 in]
          }
        }
        n127 = Select(t=T13."Enabled" ("Disabled"), s=w354, f=T13."Disabled and Grayed Out" ("Disabled")) -> (s? t:f=w353:T13)
        n128 = property on="Temp chart" class="WFChart (strict)"("DisabledEnum"=w353) -> ()  [unwired: 2 in, 2 out]
      }
      event "Instrument on/off.K-6430": Value Change {
        n129 = event-data() -> ("NewVal"=w382:bool)  [unwired: 1 in]
        n130 = case shown="False" w382 {
          selector: w382 -> [w395 w405]
          tunnel: w391 -> [w399 _]
          tunnel: [w394 w404] -> w390
          frame False {
            n131 = Unbundle(w399) -> ("Keithley-6430"=w398:refnum<visa-resource-name>, "error out"=w397:errorcluster)  [unwired: 1 out]
            n132 = call "Enable Output.vi"("error in (no error)"=w397, "Enable Output (F:Off)"=FALSE ("Output (F:Off)"), "VISA resource name"=w398) -> ("error out"=w400:errorcluster, "VISA resource name out"=w401:refnum<visa-resource-name>)  [unwired: 7 out]
            n133 = call "Close.vi"("error in (no error)"=w400, "VISA resource name"=w401) -> ("error out"=w392:errorcluster)  [unwired: 9 out]
            n134 = call <vilib>:"Simple Error Handler.vi"("error in (no error)"=w392) -> ("error out"=w396:errorcluster)  [unwired: 4 in, 4 out]
            n135 = Bundle("VISA resource name out"=refnum<visa-resource-name> refnum, "error out"=w396, w395) -> (w394:T35)  [unwired: 1 in]
          }
          frame True {
            w408 = u16 0 items=["DC Volts", "DC Current"] ("Source Function (0: DC Volts)")
            w414 = u16 0 items=["On", "Off", "Once"] ("Autozero  (0: On)")
            w420 = TRUE  # Output (F:Off)
            n136 = call "Initialize.vi"("VISA resource name"=refnum<visa-resource-name> "GPIB0::30::INSTR") -> ("error out"=w415:errorcluster, "VISA resource name out"=w416:refnum<visa-resource-name>)  [unwired: 4 in, 5 out]
            n137 = call "Configure Autozero.vi"("error in (no error)"=w415, "Autozero  (0: On)"=w414, "VISA resource name"=w416) -> ("error out"=w411:errorcluster, "VISA resource name out"=w413:refnum<visa-resource-name>)  [unwired: 7 in]
            n138 = call "Configure Source.vi"("I-Source Level [A]"=1e-09, "error in (no error)"=w411, "Auto Range (T:Enable)"=TRUE, "Source Function (0: DC Volts)"=w408, "VISA resource name"=w413) -> ("error out"=w410:errorcluster, "VISA resource name out"=w412:refnum<visa-resource-name>)  [unwired: 5 in]
            n139 = call "Configure MeasureOhms.vi"("error in (no error)"=w410, "Auto Range (T:Enable)"=TRUE, "VISA resource name"=w412) -> ("error out"=w421:errorcluster, "VISA resource name out"=w419:refnum<visa-resource-name>)  [unwired: 3 in, 4 out]
            n140 = call "Enable Output.vi"("error in (no error)"=w421, "Enable Output (F:Off)"=w420, "VISA resource name"=w419) -> ("error out"=w403:errorcluster, "VISA resource name out"=w406:refnum<visa-resource-name>)  [unwired: 7 out]
            n141 = Bundle("VISA resource name out"=w406, "error out"=w403, w405) -> (w404:T35)  [unwired: 1 in]
          }
        }
        n142 = Select(t=T13."Enabled" ("Disabled"), s=w382, f=T13."Disabled and Grayed Out" ("Disabled")) -> (s? t:f=w379:T13)
        n143 = property on="K-6430 Ohms" class="WFChart (strict)"("DisabledEnum"=w379) -> ()  [unwired: 2 in, 2 out]
      }
      event "Instrument on/off.K-2420": Value Change {
        n144 = event-data() -> ("NewVal"=w423:bool)  [unwired: 1 in]
        n145 = case shown="True" w423 {
          selector: w423 -> [w438 w448]
          tunnel: [w436 w447] -> w434
          tunnel: w433 -> [w442 _]
          frame False {
            n146 = Unbundle(w442) -> ("Keithley-2420"=w441:refnum<visa-resource-name>, "error out"=w440:errorcluster)  [unwired: 1 out]
            n147 = call "Enable Output.vi"("error in (no error)"=w440, "Enable Output (T: Enable)"=FALSE, "VISA resource name"=w441) -> ("error out"=w445:errorcluster, "VISA resource name out"=w443:refnum<visa-resource-name>)  [unwired: 7 in]
            n148 = call "Close.vi"("error in (no error)"=w445, "VISA resource name"=w443) -> ("error out"=w439:errorcluster)  [unwired: 9 in]
            n149 = call <vilib>:"Simple Error Handler.vi"("error in (no error)"=w439) -> ("error out"=w435:errorcluster)  [unwired: 4 in, 4 out]
            n150 = Bundle("VISA resource name out"=refnum<visa-resource-name> refnum, "error out"=w435, w438) -> (w436:T35)  [unwired: 1 in]
          }
          frame True {
            w456 = u16 0 items=["Voltage", "Current"] ("Source Mode  (0: Voltage)")
            w451 = u16 2 items=["Volts", "Current", "Resistance"] ("Function (0: Volts)")
            n151 = call "Initialize.vi"("VISA resource name"=refnum<visa-resource-name> "GPIB1::24::INSTR") -> ("error out"=w461:errorcluster, "VISA resource name out"=w458:refnum<visa-resource-name>)  [unwired: 9 in]
            n152 = call "Enable Remote Sensing.vi"("error in (no error)"=w461, "Enable Remote Sensing (T: Enable)"=FALSE ("4-wire?"), "VISA resource name"=w458) -> ("error out"=w460:errorcluster, "VISA resource name out"=w459:refnum<visa-resource-name>)  [unwired: 7 in]
            n153 = call "Configure Measurement.vi"("error in (no error)"=w460, "Enable Auto Range (T:Enable)"=TRUE, "Function (0: Volts)"=w451, "VISA resource name"=w459) -> ("error out"=w452:errorcluster, "VISA resource name out"=w453:refnum<visa-resource-name>)  [unwired: 6 in]
            n154 = call "Configure Output.vi"("Source Mode  (0: Voltage)"=w456, "error in (no error)"=w452, "Output Level (0)"=0.01 ("Applied Voltage (V)"), "VISA resource name"=w453) -> ("error out"=w454:errorcluster, "VISA resource name out"=w455:refnum<visa-resource-name>)  [unwired: 6 in]
            n155 = call "Enable Output.vi"("error in (no error)"=w454, "VISA resource name"=w455) -> ("error out"=w446:errorcluster, "VISA resource name out"=w449:refnum<visa-resource-name>)  [unwired: 8 in]
            n156 = Bundle("VISA resource name out"=w449, "error out"=w446, w448) -> (w447:T35)  [unwired: 1 in]
          }
        }
        n157 = Select(t=T13."Enabled" ("Disabled"), s=w423, f=T13."Disabled and Grayed Out" ("Disabled")) -> (s? t:f=w422:T13)
        n158 = property on="K-2420 Ohms" class="WFChart (strict)"("DisabledEnum"=w422) -> ()  [unwired: 2 in, 2 out]
      }
      event "Instrument on/off.K-2100": Value Change {
        n159 = event-data() -> ("NewVal"=w465:bool)  [unwired: 1 in]
        n160 = case shown="False" w465 {
          selector: w465 -> [w480 w486]
          tunnel: w475 -> [w483 _]
          tunnel: [w479 w485] -> w474
          frame False {
            n161 = Unbundle(w483) -> ("Keithley-2100"=w482:refnum<visa-resource-name>, "error out"=w481:errorcluster)  [unwired: 1 out]
            n162 = call "Close.vi"("VISA resource name"=w482, "error in (no error)"=w481) -> ("error out"=w477:errorcluster)  [unwired: 17 in]
            n163 = call <vilib>:"Simple Error Handler.vi"("error in (no error)"=w477) -> ("error out"=w476:errorcluster)  [unwired: 4 in, 4 out]
            n164 = Bundle("VISA resource name out"=refnum<visa-resource-name> refnum, "error out"=w476, w480) -> (w479:T35)  [unwired: 1 in]
          }
          frame True {
            n165 = call "Initialize.vi"("VISA resource name"=refnum<visa-resource-name> "K-2100", "Reset? (T: Reset)"=FALSE) -> ("VISA resource name out"=w490:refnum<visa-resource-name>, "error out"=w491:errorcluster)  [unwired: 16 in]
            n166 = call-poly "Configure Measurement.vi"("VISA resource name"=w490, "error in (no error)"=w491) -> ("VISA resource name out"=w487:refnum<visa-resource-name>, "error out"=w484:errorcluster)  [unwired: 16 in]
            n167 = Bundle("VISA resource name out"=w487, "error out"=w484, w486) -> (w485:T35)  [unwired: 1 in]
          }
        }
        n168 = Select(t=T13."Enabled" ("Disabled"), s=w465, f=T13."Disabled and Grayed Out" ("Disabled")) -> (s? t:f=w464:T13)
        n169 = property on="K-2100 Ohms" class="WFChart (strict)"("DisabledEnum"=w464) -> ()  [unwired: 2 in, 2 out]
      }
      event "Instrument on/off.SRS QCM": Value Change {
        n170 = event-data() -> ("NewVal"=w492:bool)  [unwired: 1 in]
        n171 = case shown="False" w492 {
          selector: w492 -> [w507 w515]
          tunnel: w504 -> [w511 w516]
          tunnel: [w508 w513] -> w503
          frame False {
            n172 = Unbundle(w511) -> ("SRS-QCM200"=w510:refnum<visa-resource-name>, "error out"=w505:errorcluster)  [unwired: 1 out]
            n173 = call "srsQcm200Close.vi"("error in"=w505, "Visa in"=w510) -> ("error out"=w509:errorcluster)  [unwired: 3 in]
            n174 = Bundle("VISA resource name out"=refnum<visa-resource-name> refnum, "error out"=w509, w507) -> (w508:T35)  [unwired: 1 in]
          }
          frame True {
            n175 = Unbundle(w516) -> ()  [unwired: 3 out]
            n176 = call "SrsQcm200Open.vi"("VISA in"=refnum<visa-resource-name> "COM6") -> ("error out"=w512:errorcluster, "VISA out"=w514:refnum<visa-resource-name>)  [unwired: 4 in]
            n177 = Bundle("VISA out"=w514, "error out"=w512, w515) -> (w513:T36)  [unwired: 1 in]
          }
        }
        n178 = Select(t=T13."Enabled" ("Disabled"), s=w492, f=T13."Disabled and Grayed Out" ("Disabled")) -> (s? t:f=w493:T13)
        n179 = property on="SRS cluster" class="Clust"("DisabledEnum"=w493) -> ()  [unwired: 2 in, 2 out]
      }
      event "Instrument on/off.ArduiunoQCMs": Value Change {
        n180 = event-data() -> ("NewVal"=w526:bool)  [unwired: 1 in]
        n181 = case shown="False" w526 {
          selector: w526 -> [_ w546]
          tunnel: [T24 {"arduinos on/off"=FALSE, "arduino 1-6 address and errors"={"VISA resource name out"="", "error out"={"status"=FALSE, "code"=0, "source"=""}, "VISA resource name out"="", "error out"={"status"=FALSE, "code"=0, "source"=""}, "VISA resource name out"="", "error out"={"status"=FALSE, "code"=0, "source"=""}, "VISA resource name out"="", "error out"={"status"=FALSE, "code"=0, "source"=""}, "VISA resource name out"="", "error out"={"status"=FALSE, "code"=0, "source"=""}}} w535] -> w530
          tunnel: w529 -> [w534 w544]
          frame False {
            n182 = Unbundle(w534) -> ("arduinos on/off"=w533:bool, "arduino addresses/errors"=w532:T26)
            n183 = call "arduino_close_subIV.vi"("arduino 1-6 addresses and errors out"=w532, "arduinos on?"=w533) -> ()  [unwired: 10 in]
          }
          frame True {
            n184 = Unbundle(w544) -> ("arduino addresses/errors"=w543:T26)  [unwired: 1 out]
            n185 = Unbundle(w543) -> ("VISA resource name out"=w542:refnum<visa-resource-name>, "VISA resource name out"=w541:refnum<visa-resource-name>, "VISA resource name out"=w540:refnum<visa-resource-name>, "VISA resource name out"=w539:refnum<visa-resource-name>, "VISA resource name out"=w538:refnum<visa-resource-name>)  [unwired: 5 out]
            n186 = Bundle("VISA resource name out"=w542, "VISA resource name out"=w541, "VISA resource name out"=w540, "VISA resource name out"=w539, "VISA resource name out"=w538) -> (w537:T37)  [unwired: 1 in]
            n187 = call "initialize_arduinos_subVI.vi"("arduino 1-6 addresses"=w537, "arduinos on?"=w546) -> ("arduino addresses/errors"=w536:T26, "arduinos on/off"=w545:bool)  [unwired: 8 in]
            n188 = Bundle("arduinos on/off"=w545, "arduino addresses/errors"=w536) -> (w535:T38)  [unwired: 1 in]
          }
        }
        n189 = Select(t=T13."Enabled" ("Disabled"), s=w526, f=T13."Disabled and Grayed Out" ("Disabled")) -> (s? t:f=w525:T13)
        n190 = property on="Arduino QCM plots" class="Clust (strict)"("DisabledEnum"=w525) -> ()  [unwired: 2 in, 2 out]
        n191 = property on="Arduino QCM freq" class="Clust (strict)"("DisabledEnum"=w525) -> ()  [unwired: 2 in, 2 out]
      }
    }
    n192 = Unbundle("Pressure parameters cluster") -> ("valve % open"=w103:dbl, "Desired pressure"=w104:dbl, "Vapor sccm"=w105:sgl, "Gas sccm"=w106:sgl, "Valve mode"=w107:enum32{"% Open", "Torr "}, "Pressure Mode"=w108:enum32{"Abs. pressure", " Part. pressure"}, "analyte partial pressure"=w109:dbl, "Turbo pump\nauto on"=w110:bool)  [unwired: 4 out]
    n193 = Bundle("valve % open"=w103, "Desired pressure"=w104, "Vapor sccm"=w105, "Gas sccm"=w106, "Valve mode"=w107, "Pressure Mode"=w108, "analyte partial pressure"=w109, "Turbo pump\nauto on"=w110) -> (w102:T39)  [unwired: 1 in]
    n194 = Bundle("User-defined\nsequence"=w112, "Present (s)"=w128, "current  step # in"=w125, "sequence end time in"=w126) -> (w127:T40)  [unwired: 1 in]
    n195 = call "Pressure_control_subVI _V2.vi"("Run Sequence"=w113, "user sequence, present (s) in, current step in, seq time in"=w127, "pressure parameters in"=w102, "pressure control on? / DAQ IDs/errors in"=w116) -> ("current step # out, shift register time out, seq button on?"=w124:T41, "sequence over? USE THIS TO REINITIALIZE RUN SEQUENCE BUTTON SO PROGRAM ENDS"=w118:bool, "save press/RH/gasflow/vaporflow - read valve position/pressure/vaporflow/gasflow"=w120:T42, "pressure control on out, DAQ IDs/errors out"=w115:T43, "sequence end date/time string"=w111:string)  [unwired: 3 in]
    n196 = property on="Sequence end time" class="Str"("Value"=w111) -> ()  [unwired: 2 in, 2 out]
    n197 = case shown="True" w118 {
      frame False {
      }
      frame True {
        n198 = property on="Run Sequence" class="Bool (strict)"("Value"=FALSE ("Run Sequence")) -> ()  [unwired: 2 in, 2 out]
      }
    }
    n199 = Unbundle(w120) -> ("press/RH/gas/vapor"=w119:T44, "Cluster"=w101:T45)
    n200 = Unbundle(w101) -> ("Valve position (%)"=w100:dbl, "read pressure"=w93:dbl, "read vapor flow"=w98:dbl, "read gas flow"=w99:dbl)
    "Pressure chart" <- w93
    n201 = property on="read gas flow" class="DigNum (strict)"("Value"=w99) -> ()  [unwired: 2 in, 2 out]
    n202 = property on="Valve position (%)" class="DigNum (strict)"("Value"=w100) -> ()  [unwired: 2 in, 2 out]
    n203 = property on="read pressure" class="DigNum (strict)"("Value"=w93) -> ()  [unwired: 2 in, 2 out]
    n204 = property on="read vapor flow" class="DigNum (strict)"("Value"=w98) -> ()  [unwired: 2 in, 2 out]
    n205 = Unbundle("Data logging settings") -> ("Save during sequence only"=w90:bool, "Save now"=w89:bool, "seconds between\ndata points"=w88:dbl, "Save sample names"=w83:T46, "Experiment Notes"=w84:string)  [unwired: 1 out]
    n206 = Subtract(x=w142, y=w95) -> (x-y=w170:dbl)
    n207 = And(x=w113, y=w90) -> (x .and. y?=w174:bool)
    n208 = Divide(x=w170, y=60.0) -> (x/y=w168:dbl)
    "Elapsed time (min)" <- w168
    n209 = call "data_headers_subVI_V2.vi"("Experiment Notes"=w84, "Sample names"=w83) -> ("data headers"=w182:string[])  [unwired: 9 in]
    n210 = Or(x=w174, y=w89) -> (x .or. y?=w91:bool)
    "Currently saving data" <- w91
    n211 = Get Date/Time In Seconds() -> (seconds since 1Jan1904=w185:timestamp)
    n212 = Format Date/Time String(time format string (%c)="%Y-%m-%d %H:%M:%S%2u", seconds (now)=w185) -> (date/time string=w144:string)  [unwired: 1 in]
    n213 = Number To Engineering String ("elapsed time (min)")(4:w168) -> (0:w143:string)  [unwired: 3 in]
    n214 = Multiply(x=w88, y=u32 1000 ("x")) -> (x*y=w183:dbl)
    n215 = Unbundle(w147) -> ("String data out"=w151:string, "K6430 measuremnet string"=w152:string, "String"=w153:string, "String"=w145:string)
    n216 = Unbundle(w146) -> ("mass_ug"=w148:string, "freq_Hz"=w149:string, "motional_resistance_Ohm"=w150:string)
    n217 = Unbundle(w119) -> ("pressure"=w140:string, "RH"=w139:string, "gas flow"=w138:string, "vapor flow"=w137:string)
    n218 = Unbundle ("arduino 1-6")(w129) -> ("f"=w136:string, "f"=w135:string, "f"=w134:string, "f"=w133:string, "f"=w132:string)
    n219 = Wait (ms)(milliseconds to wait=w183) -> ()  [unwired: 1 out]
    n220 = Build Array(w144, w143, w151, w152, w153, w145, w148, w149, w150, w140, w139, w138, w137, w136, w135, w134, w133, w132) -> (w141:string[])
    n221 = Unbundle(w124) -> ("current  step # in"=w123:i32, "sequence end time in"=w122:timestamp, "Boolean"=w121:bool)
    "State date/time" <- w167
  }
  n222 = Unbundle(w25) -> ("DAQ IDs in"=w24:T47)  [unwired: 1 out]
  n223 = call-poly <vilib>:"Write To Spreadsheet File.vi"("1D data"=w63, "file path (dialog if empty)"=w65) -> ("new file path (Not A Path if cancelled)"=w68:path)  [unwired: 6 in]
  n224 = Unbundle(w24) -> ("task out"=w43:refnum<k21>, "error out"=w44:errorcluster, "task out"=w45:refnum<k21>, "error out"=w46:errorcluster, "task out"=w47:refnum<k21>, "error out"=w48:errorcluster, "VISA Refnum out"=w49:refnum<visa-resource-name>, "error out"=w50:errorcluster)
  n225 = call-poly <vilib>:"Write To Spreadsheet File.vi"("append to file? (new file:F)"=TRUE, "2D data"=w58, "file path (dialog if empty)"=w68) -> ()  [unwired: 5 in, 1 out]
  n226 = disable-structure shown="Disabled" {
    disable-tunnel: [w549 _] -> w51
    disable-tunnel: w43 -> [w548 _]
    disable-tunnel: w44 -> [w547 _]
    frame Disabled {
      n227 = call <vilib>:"DAQmx Stop Task.vi"("task/channels in"=w548, "error in"=w547) -> ("task out"=w550:refnum<k21>, "error out"=w551:errorcluster)  [unwired: 12 in]
      n228 = call <vilib>:"DAQmx Clear Task.vi"("task in"=w550, "error in"=w551) -> ("error out"=w549:errorcluster)  [unwired: 13 in]
    }
    frame Enabled {
    }
  }
  n229 = call <vilib>:"DAQmx Stop Task.vi"("task/channels in"=w45, "error in"=w46) -> ("task out"=w39:refnum<k21>, "error out"=w40:errorcluster)  [unwired: 12 in]
  n230 = call <vilib>:"DAQmx Stop Task.vi"("task/channels in"=w47, "error in"=w48) -> ("task out"=w38:refnum<k21>, "error out"=w37:errorcluster)  [unwired: 12 in]
  n231 = VISA Clear(VISA resource name=w49, error in (no error)=w50) -> (VISA resource name out=w41:refnum<visa-resource-name>, error out=w42:errorcluster)
  n232 = VISA Close(VISA resource name=w41, error in (no error)=w42) -> (error out=w54:errorcluster)
  n233 = call <vilib>:"DAQmx Clear Task.vi"("task in"=w39, "error in"=w40) -> ("error out"=w52:errorcluster)  [unwired: 13 in]
  n234 = call <vilib>:"DAQmx Clear Task.vi"("task in"=w38, "error in"=w37) -> ("error out"=w53:errorcluster)  [unwired: 13 in]
  n235 = Merge Errors(w51, w52, w53, w54) -> (w55:errorcluster)
  n236 = call <vilib>:"Simple Error Handler.vi"("error in (no error)"=w55) -> ()  [unwired: 4 in, 5 out]
